vi "DHE_GetModifiersInfo.vi"(8 "error in (no error)":errorcluster) -> (0 "error out":errorcluster, 1 "xpost":i32, 2 "modifiers":string, 3 "xpre":i32, 4 "Binning.y":u32, 5 "ypre":i32, 6 "Binning.x":u32, 7 "ypost":i32)   [LabVIEW 2016]
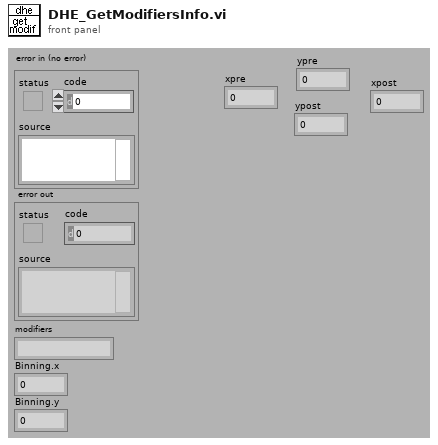
[diagram p1: front panel]
types:
  T1 = typedef "GEOM_AmpModifiers.ctl" = cluster{"Binning":T2, "sections":T3[]}
  T2 = typedef "GEOM_Binning.ctl" = cluster{"x":u32, "y":u32}
  T3 = typedef "GEOM_Moifier.ctl" = cluster{"name":string, "header section":string, "comment":string, "value":i32, "binning?":bool, "Where":enum16{"predata", "postdata"}, "add In":enum16{"columns", "rows", "none"}}
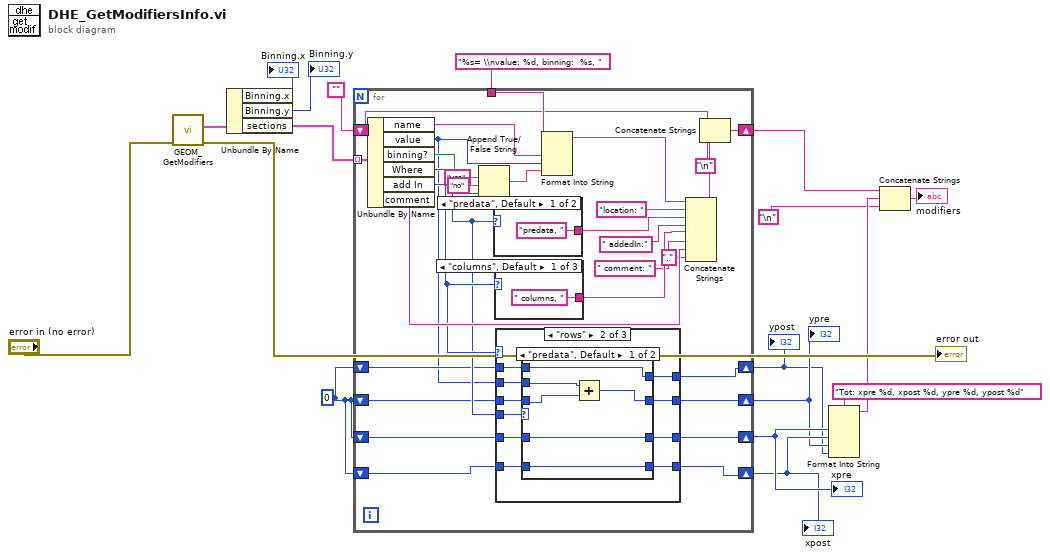
[diagram p0: block diagram]
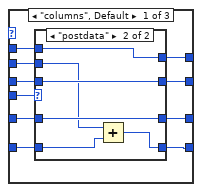
[diagram p2: hidden frame]
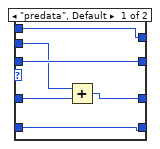
[diagram p3: hidden frame]
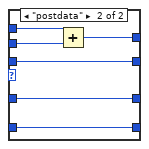
[diagram p4: hidden frame]
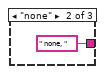
[diagram p6: hidden frame]
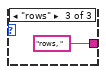
[diagram p7: hidden frame]
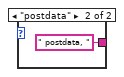
[diagram p8: hidden frame]
diagram:
  w12 = 0
  n1 = call "GEOM_GetModifiers.vi"("error in (no error)"="error in (no error)") -> ("error out"=→"error out":errorcluster, "GEOM_modifiers"=w17:T1)  [unwired: 9 out]
  n2 = Unbundle By Name(w17) -> ("Binning.x"=→"Binning.x":u32, "Binning.y"=→"Binning.y":u32, "sections"=w16:T3[])
  n3 = for {
    tunnel: w16 -> [w48] mode=indexing
    tunnel: "%s= \\nvalue: %d, binning:  %s, " ("format string") -> [w47]
    shift-right: [w36] -> w11
    shift-left: "" -> [w35]
    shift-right: [w19] -> w1
    shift-left: w12 -> [w21]
    shift-right: [w22] -> w2
    shift-left: w12 -> [w23]
    shift-right: [w24] -> w9
    shift-left: w12 -> [w25]
    shift-right: [w26] -> w8
    shift-left: w12 -> [w27]
    n4 = Unbundle By Name(w48) -> ("name"=w46:string, "value"=w20:i32, "binning?"=w33:bool, "Where"=w28:enum16{"predata", "postdata"}, "add In"=w29:enum16{"columns", "rows", "none"}, "comment"=w39:string)
    n5 = Append True/False String(1:w33, 2:"no" ("false string"), 3:"yes" ("true string")) -> (0:w30:string)  [unwired: 1 out]
    n6 = case shown="\"predata\", Default" w28 {
      tunnel: ["predata, " " postdata, "] -> w43
      frame "predata", Default {
      }
      frame "postdata" {
      }
    }
    n7 = case shown="\"columns\", Default" w29 {
      tunnel: [" columns, " " none, " "rows, "] -> w41
      frame "columns", Default {
      }
      frame "none" {
      }
      frame "rows" {
      }
    }
    n8 = case shown="\"rows\"" w29 {
      tunnel: w28 -> [w58 w80 _]
      tunnel: w27 -> [w57 w79 w93]
      tunnel: [w49 w78 w93] -> w26
      tunnel: w25 -> [w56 w77 w94]
      tunnel: [w55 w76 w94] -> w24
      tunnel: w23 -> [w54 w75 w95]
      tunnel: [w53 w74 w95] -> w22
      tunnel: w21 -> [w52 w73 w96]
      tunnel: w20 -> [w51 w72 _]
      tunnel: [w50 w71 w96] -> w19
      frame "columns", Default {
        n9 = case shown="\"postdata\"" w58 {
          tunnel: w57 -> [w59 w66]
          tunnel: w56 -> [w62 w70]
          tunnel: [w60 w70] -> w55
          tunnel: [w63 w69] -> w53
          tunnel: w54 -> [w63 w69]
          tunnel: w52 -> [w64 w68]
          tunnel: w51 -> [w61 w67]
          tunnel: [w64 w68] -> w50
          tunnel: [w59 w65] -> w49
          frame "predata", Default {
            n10 = Add(x=w61, y=w62) -> (x+y=w60:i32)
          }
          frame "postdata" {
            n11 = Add(x=w67, y=w66) -> (x+y=w65:i32)
          }
        }
      }
      frame "rows" {
        n12 = case shown="\"predata\", Default" w80 {
          tunnel: [w81 w92] -> w78
          tunnel: w79 -> [w81 w92]
          tunnel: w77 -> [w82 w91]
          tunnel: [w82 w91] -> w76
          tunnel: [w83 w90] -> w74
          tunnel: w75 -> [w84 w90]
          tunnel: w73 -> [w86 w89]
          tunnel: w72 -> [w85 w88]
          tunnel: [w86 w87] -> w71
          frame "predata", Default {
            n13 = Add(x=w85, y=w84) -> (x+y=w83:i32)
          }
          frame "postdata" {
            n14 = Add(x=w89, y=w88) -> (x+y=w87:i32)
          }
        }
      }
      frame "none" {
      }
    }
    n15 = Format Into String(format string=w47, w46, w20, w30) -> (resulting string=w45:string)  [unwired: 2 in, 1 out]
    n16 = Concatenate Strings(w45, "location: ", w43, " addedIn:", w41, " comment: " ("string"), w39, "." ("string")) -> (w38:string)
    n17 = Concatenate Strings(w35, w38, "\n") -> (w36:string)
  }
  "ypost" <- w1
  "ypre" <- w2
  "xpre" <- w9
  "xpost" <- w8
  n18 = Format Into String(format string="Tot: xpre %d, xpost %d, ypre %d, ypost %d", w9, w8, w2, w1) -> (resulting string=w7:string)  [unwired: 2 in, 1 out]
  n19 = Concatenate Strings(w11, w7, "\n") -> (→"modifiers":string)
